vi "array_to_string.vi"(1 "Real Matrix":dbl[](array[numeric])) -> (0 "String":string)   [LabVIEW 2019]
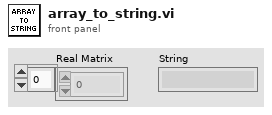
[diagram p1: front panel]
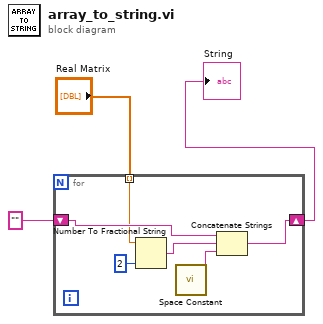
[diagram p0: block diagram]
diagram:
  n1 = for {
    shift-right: [w5] -> w3
    shift-left: "" -> [w6]
    tunnel: "Real Matrix" -> [w4] mode=indexing
    n2 = Number To Fractional String(number=w4, precision (6)=i16 2) -> (F-format string=w8:string)  [unwired: 2 in]
    n3 = call <vilib>:"Space Constant.vi"() -> ("String"=w7:string)
    n4 = Concatenate Strings(w6, w8, w7) -> (w5:string)
  }
  "String" <- w3
